vi "Close.vi"(8 "error in":errorcluster, 11 "Config from EXCEL in":refnum<class "Config from EXCEL.lvclass">) -> (0 "error out":errorcluster, 3 "Config from EXCEL out":refnum<class "Config from EXCEL.lvclass">)   [LabVIEW 2024, in "Config from EXCEL.lvclass"]
uses:
  Config from EXCEL.lvclass
  Config from EXCEL.lvclass/Config from EXCEL.ctl
  Open-Xml-LabVIEW/Source/Open Xml.lvlib
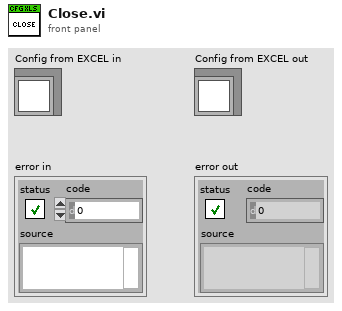
[diagram p1: front panel]
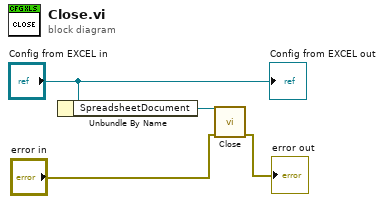
[diagram p0: block diagram]
diagram:
  n1 = Unbundle By Name("Config from EXCEL in") -> ("SpreadsheetDocument"=w3:refnum<k24>)
  n2 = call "Close.vi"("error in"="error in", "SpreadsheetDocument"=w3) -> ("error out"=→"error out":errorcluster)  [unwired: 9 in]
  "Config from EXCEL out" <- "Config from EXCEL in"
